vi "Build Major Frame Definition.vi"(8 "error in (no error)":errorcluster, 11 "Bus Controller XML Node":refnum<k20>) -> (0 "error out":errorcluster, 1 "Major Schedule":refnum<queue>, 2 "Minor Frame Rate":u16, 5 "Major Frame ID":string)   [LabVIEW 2016]
doc: "Reads the Major Frame node from XML to generate the sequence that is used for building the Major Frame. Additionally retrieves the Major Frame ID and Minor Frame rate in use in this Major Frame."
uses:
  <vilib>/xml/NI_XML.lvlib
  <resource>/objmgr/DOMUserDefRef.rc
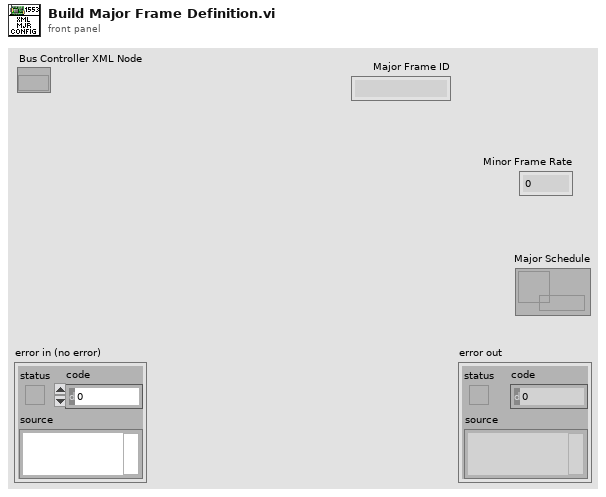
[diagram p1: front panel]
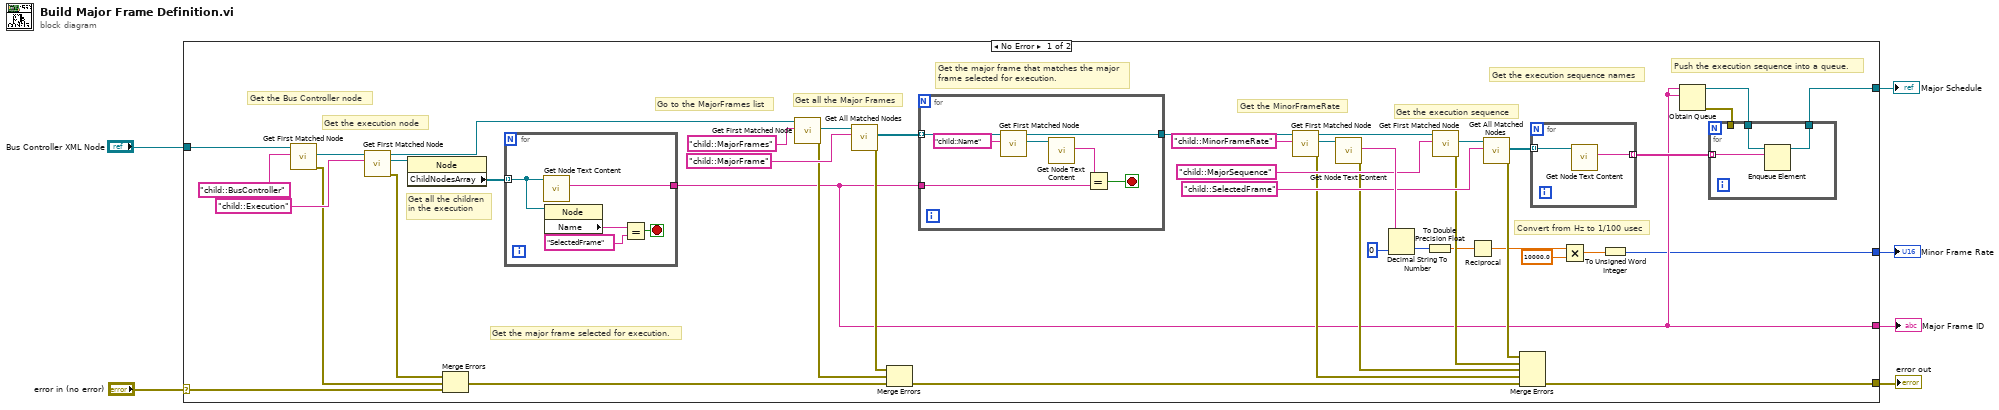
[diagram p0: block diagram]
diagram:
  n1 = case shown="No Error" "error in (no error)" {
    selector: "error in (no error)" -> [w40 w68]
    tunnel: [w19 w68] -> w5
    tunnel: "Bus Controller XML Node" -> [w50 _]
    tunnel: [w43 _] -> w3
    tunnel: [w13 _] -> w2
    tunnel: [w7 _] -> w1
    frame No Error {
      # "Convert from Hz to 1/100 usec"
      # "Get the execution sequence names"
      # "Push the execution sequence into a queue."
      # "Get the execution sequence"
      # "Get the MinorFrameRate"
      # "Get the major frame that matches the major\nframe selected for execution."
      # "Get all the Major Frames"
      # "Go to the MajorFrames list"
      # "Get the major frame selected for execution."
      # "Get all the children\nin the execution"
      # "Get the execution node"
      # "Get the Bus Controller node"
      n2 = call <vilib>:"Get First Matched Node.vi"("XPath expression"="child::BusController", "node in"=w50) -> ("error out"=w41:errorcluster, "node result"=w48:refnum<k20>)  [unwired: 7 in, 1 out]
      n3 = call <vilib>:"Get First Matched Node.vi"("XPath expression"="child::Execution", "node in"=w48) -> ("error out"=w42:errorcluster, "node result"=w46:refnum<k20>, "node out"=w38:refnum<k20>)  [unwired: 7 in]
      n4 = property class="Node"(reference=w46) -> ("ChildNodesArray"=w45:refnum<k20>[])  [unwired: 1 in, 2 out]
      n5 = Merge Errors(w42, w41, w40) -> (w23:errorcluster)
      n6 = for {
        tunnel: w45 -> [w66] mode=indexing
        tunnel: [w67] -> w13
        stop <- w63 stop-if-true
        n7 = call <vilib>:"Get Node Text Content.vi"("node in"=w66) -> ("node text"=w67:string)  [unwired: 8 in, 2 out]
        n8 = property class="Node"(reference=w66) -> ("Name"=w65:string)  [unwired: 1 in, 2 out]
        n9 = Equal?(x=w65, y="SelectedFrame") -> (x = y?=w63:bool)
      }
      n10 = call <vilib>:"Get First Matched Node.vi"("XPath expression"="child::MajorFrames", "node in"=w38) -> ("error out"=w22:errorcluster, "node result"=w36:refnum<k20>)  [unwired: 7 in, 1 out]
      n11 = call <vilib>:"Get All Matched Nodes.vi"("XPath expression"="child::MajorFrame", "node in"=w36) -> ("error out"=w21:errorcluster, "node result array"=w34:refnum<k20>[])  [unwired: 7 in, 1 out]
      n12 = Merge Errors(w21, w22, w23) -> (w20:errorcluster)
      n13 = for {
        tunnel: w34 -> [w59] mode=indexing
        tunnel: w13 -> [w55]
        tunnel: [w54] -> w32
        stop <- w53 stop-if-true
        n14 = call <vilib>:"Get First Matched Node.vi"("XPath expression"="child::Name", "node in"=w59) -> ("node result"=w57:refnum<k20>, "node out"=w54:refnum<k20>)  [unwired: 7 in, 1 out]
        n15 = call <vilib>:"Get Node Text Content.vi"("node in"=w57) -> ("node text"=w56:string)  [unwired: 8 in, 2 out]
        n16 = Equal?(x=w56, y=w55) -> (x = y?=w53:bool)
      }
      n17 = call <vilib>:"Get First Matched Node.vi"("XPath expression"="child::MinorFrameRate", "node in"=w32) -> ("error out"=w18:errorcluster, "node result"=w31:refnum<k20>, "node out"=w28:refnum<k20>)  [unwired: 7 in]
      n18 = call <vilib>:"Get Node Text Content.vi"("node in"=w31) -> ("error out"=w17:errorcluster, "node text"=w30:string)  [unwired: 8 in, 1 out]
      n19 = Decimal String To Number(string=w30, default (0L)=u16 0 ("Minor Frame Rate")) -> (number=w12:u16)  [unwired: 1 in, 1 out]
      n20 = To Double Precision Float(number=w12) -> (double precision float=w11:dbl)
      n21 = call <vilib>:"Get First Matched Node.vi"("XPath expression"="child::MajorSequence", "node in"=w28) -> ("error out"=w16:errorcluster, "node result"=w26:refnum<k20>)  [unwired: 7 in, 1 out]
      n22 = Reciprocal(x=w11) -> (1/x=w10:dbl)
      n23 = call <vilib>:"Get All Matched Nodes.vi"("XPath expression"="child::SelectedFrame", "node in"=w26) -> ("error out"=w15:errorcluster, "node result array"=w24:refnum<k20>[])  [unwired: 7 in, 1 out]
      n24 = Merge Errors(w15, w16, w17, w18, w20) -> (w19:errorcluster)
      n25 = for {
        tunnel: w24 -> [w52] mode=indexing
        tunnel: [w51] -> w14 mode=indexing
        n26 = call <vilib>:"Get Node Text Content.vi"("node in"=w52) -> ("node text"=w51:string)  [unwired: 8 in, 2 out]
      }
      n27 = Multiply(x=w10, y=10000.0) -> (x*y=w8:dbl)
      n28 = To Unsigned Word Integer(number=w8) -> (unsigned 16bit integer=w7:u16)
      n29 = Obtain Queue(name (unnamed)=w13, element data type=w13) -> (queue out=w44:refnum<queue>, error out=w39:errorcluster)  [unwired: 3 in, 1 out]
      n30 = for {
        tunnel: w44 -> [w62]
        tunnel: [w61] -> w43
        tunnel: w39 -> [_]
        tunnel: w14 -> [w60] mode=indexing
        n31 = Enqueue Element(queue=w62, element=w60) -> (queue out=w61:refnum<queue>)  [unwired: 2 in, 2 out]
      }
    }
    frame Error {
    }
  }
  "error out" <- w5
  "Major Schedule" <- w3
  "Major Frame ID" <- w2
  "Minor Frame Rate" <- w1
